vi "fgm_pipeline_partial_N22.vi"(6 "du_max":fxp<+/-,18,1>, 8 "x_vec":T3=[0.0, 0.0, 0.0, 0.0, 0.0, 0.0, 0.0, 0.0, 0.0, 0.0, 0.0, 0.0, 0.0, 0.0, 0.0, 0.0, 0.0, 0.0, 0.0, 0.0, 0.0, 0.0, 0.0, 0.0, 0.0], 11 "QP_params":T4={"maxIter"=0, "nuN"=24, "Ns_mpc"=0, "-beta"=-0.9987945556640625, "beta+1"=1.9987945556640625}) -> (0 "z":T1, 1 "delta u(k)":fxp<+/-,32,3>, 4 "y":T1)   [LabVIEW 2017]
uses:
  quadProgParams_pipe.ctl
  x_vec_type_pipe.ctl
  x_qp_scalar.ctl
  ziyi_pipe.ctl
  xtype_scalar.ctl
  <vilib>/rvi/Emulation/niFpgaEmulationIsFPGAContextNoSignature.vi
  <vilib>/rvi/DataTransferAndStorage/Container/Common/niFpgaContainerGetUniqueNameForEmu.vi
  <vilib>/rvi/Memory/Memory_Emulation/niFpgaMemoryEmulationCacheClearOnFirstRun.vi
  <vilib>/rvi/Memory/Memory_Emulation/nirvimemoryEmulationManagerCache_MakeExclusive.vi
  <vilib>/rvi/Memory/Memory_Emulation/niFpgaMemoryEmulationValidateCache.vi
  <vilib>/rvi/Memory/Memory_Emulation/nirvimemoryEmulationManagerCache_InsertValue.vi
  <vilib>/Utility/error.llb/Clear Errors.vi
  <vilib>/rvi/Memory/Memory_Emulation/nirvimemoryEmulationManagerCache_ReleaseExclusive.vi
  <vilib>/rvi/Memory/Memory_Emulation/nirvimemoryEmulationManagerCache_GetValue.vi
  <vilib>/rvi/Memory/Memory_Emulation/nirvimemoryEmulationManagerCache_SetValue.vi
  <vilib>/rvi/Emulation/niFpgaProcessEmulError.vi
  <vilib>/rvi/Emulation/niFpgaSctlEmulationGetInTimedLoop.vi
  <vilib>/rvi/DataTransferAndStorage/Container/XNode/niFpgaContainer.xnode
  <vilib>/rvi/DataTransferAndStorage/Register/Emulation/niFpgaRegisterEmulation.vi
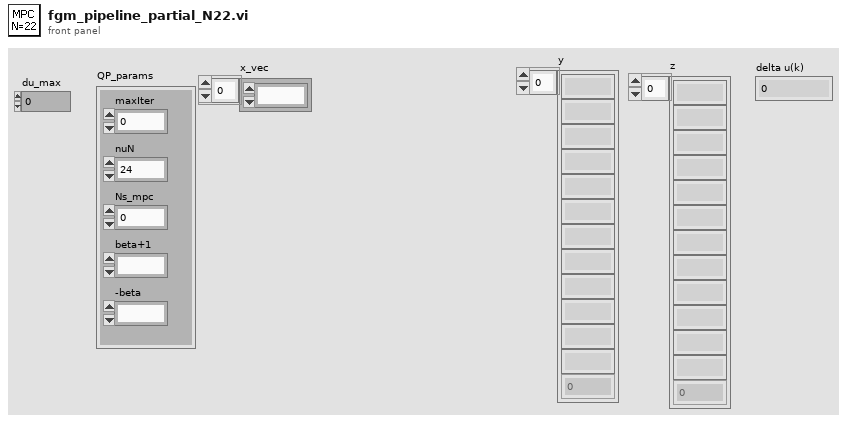
[diagram p1: front panel]
types:
  T1 = typedef "ziyi_pipe.ctl" = T2[]
  T2 = typedef "x_qp_scalar.ctl" = fxp<+/-,32,6>
  T3 = typedef "x_vec_type_pipe.ctl" = T2[]
  T4 = typedef "quadProgParams_pipe.ctl" = cluster{"maxIter":u16, "nuN":u16, "Ns_mpc":u16, "-beta":fxp<+/-,18,2>, "beta+1":fxp<+/-,18,2>}
  T5 = typedef "xtype_scalar.ctl" = fxp<+/-,32,6>
  T6 = typedef "ziyi_pipe_N22.ctl" = T2[]
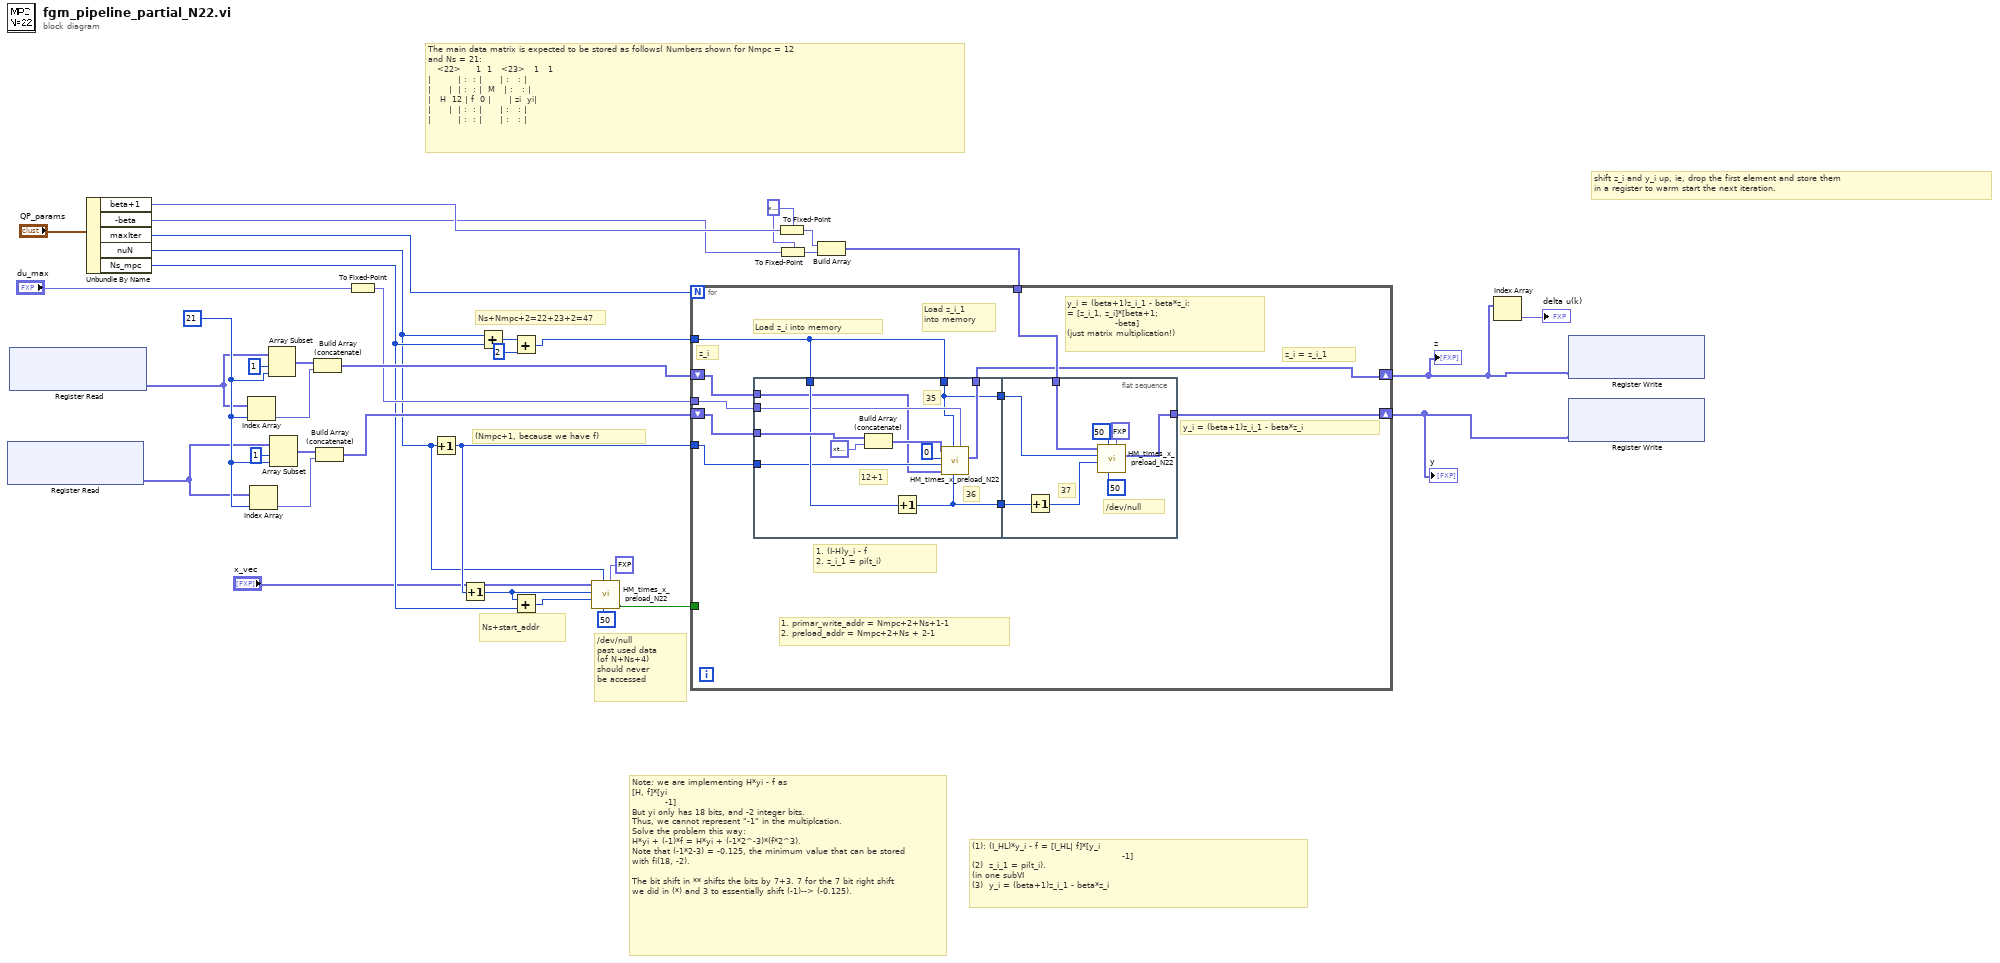
[diagram p0: block diagram]
diagram:
  w12 = 21 ("length")
  w19 = T5 0.0 ("xtype")
  # "The main data matrix is expected to be stored as follows( Numbers shown for Nmpc = 12\nand Ns = 21:\n   <22>     1  1   <23>   1   1\n|         | :  : |      | :   : |\n|      |  | :  : |  M   | :   : |\n|   H  12 | f  0 |      | zi  yi|\n|      |  | :  : |      | :   : |\n|         | :  : |      | :   : |"
  # "Ns+Nmpc+2=22+23+2=47"
  # "Ns+start_addr"
  # "(Nmpc+1, because we have f)"
  # "/dev/null\npast used data\n(of N+Ns+4)\nshould never\nbe accessed"
  # "Note: we are implementing H*yi - f as\n[H, f]*[yi\n           -1]\nBut yi only has 18 bits, and -2 integer bits. \nThus, we cannot represent \"-1\" in the multiplcation.\nSolve the problem this way:\nH*yi + (-1)*f = H*yi + (-1*2^-3)*(f*2^3).\nNote that (-1*2-3) = -0.125, the minimum value that can be stored\nwith fi(18, -2).\n\nThe bit shift in ** shifts the bits by 7+3. 7 for the 7 bit right shift\nwe did in (*) and 3 to essentially shift (-1)--> (-0.125)."
  # "(1): (I_HL)*y_i - f = [I_HL| f]*[y_i\n                                                  -1]\n(2)  z_i_1 = pi(t_i).\n(in one subVI\n(3)  y_i = (beta+1)z_i_1 - beta*z_i"
  # "shift z_i and y_i up, ie, drop the first element and store them\nin a register to warm start the next iteration."
  n1 = xnode ("Register Read")() -> ("Data"=w9:fxp<+/-,32,6>[])  [unwired: 1 in, 1 out]
  n2 = xnode ("Register Read")() -> ("Data"=w8:fxp<+/-,32,6>[])  [unwired: 1 in, 1 out]
  n3 = Unbundle By Name("QP_params") -> ("beta+1"=w34:fxp<+/-,18,2>, "-beta"=w33:fxp<+/-,18,2>, "maxIter"=w35:u16, "nuN"=w7:u16, "Ns_mpc"=w16:u16)
  n4 = Index Array(array=w8, index=w12) -> (element=w22:fxp<+/-,32,6>)
  n5 = Index Array(array=w9, index=w12) -> (element=w23:fxp<+/-,32,6>)
  n6 = Array Subset(array=w8, index=1, length=w12) -> (w26:fxp<+/-,32,6>[])
  n7 = Array Subset(array=w9, index=1, length=w12) -> (w24:fxp<+/-,32,6>[])
  n8 = Build Array (concatenate)(w26, w22) -> (w21:fxp<+/-,32,6>[])
  n9 = Build Array (concatenate)(w24, w23) -> (w20:fxp<+/-,32,6>[])
  n10 = To Fixed-Point(number="du_max") -> (fixed-point=w18:fxp<+/-,18,5>)  [unwired: 1 in]
  n11 = Increment(x=w7) -> (x+1=w29:u16)
  n12 = Increment(x=w29) -> (x+1=w2:u16)
  n13 = Add(x=w7, y=w16) -> (x+y=w15:u16)
  n14 = Add(x=w15, y=u16 2) -> (x+y=w13:u16)
  n15 = Add(x=w2, y=w16) -> (x+y=w1:u16)
  n16 = call "HM_times_x_preload_N22.vi"("SLMAX"=fxp<+/-,18,5> 15.9998779296875, "preload_addr"=u8 50, "primary_write_addr"=w7, "Ns+StartIndex"=w1, "StartIndex"=w2, "x_vec"="x_vec") -> ("done"=w5:bool)  [unwired: 4 in, 1 out]
  n17 = To Fixed-Point(fixed-point type=w19, number=w34) -> (fixed-point=w32:T5)
  n18 = To Fixed-Point(fixed-point type=w19, number=w33) -> (fixed-point=w31:T5)
  n19 = Build Array(w32, w31) -> (w30:T5[])
  n20 = for {
    N: w35 -> [_]
    shift-right: [w45] -> w10
    shift-left: w20 -> [w44]
    shift-right: [w41] -> w11
    shift-left: w21 -> [w40]
    tunnel: w30 -> [w46]
    tunnel: w18 -> [w42]
    tunnel: w5 -> [_]
    tunnel: w29 -> [w43]
    tunnel: w13 -> [w38]
    # "1. primar_write_addr = Nmpc+2+Ns+1-1\n2. preload_addr = Nmpc+2+Ns + 2-1"
    # "y_i = (beta+1)z_i_1 - beta*z_i:\n= [z_i_1, z_i]*[beta+1;\n                -beta]\n(just matrix multiplication!)"
    # "Load z_i into memory"
    # "Load z_i_1\ninto memory"
    # "1. (I-H)y_i - f\n2. z_i_1 = pi(t_i)"
    # "z_i = z_i_1"
    # "y_i = (beta+1)z_i_1 - beta*z_i"
    # "z_i"
    n21 = flat-sequence {
      tunnel: w40 -> [w47]
      tunnel: w44 -> [w57]
      tunnel: w43 -> [w48]
      tunnel: w42 -> [w52]
      tunnel: [w53] -> w41
      tunnel: w38 -> [w51]
      tunnel: [w51] -> w39
      tunnel: w38 -> [w55]
      tunnel: [w50] -> w37
      tunnel: w46 -> [w60]
      tunnel: [w64] -> w45
      tunnel: w39 -> [w61]
      tunnel: w37 -> [w65]
      frame #0 {
        # "35"
        # "36"
        # "12+1"
        n22 = Build Array (concatenate)(w57, T5 -1.0 ("xtype")) -> (w54:T5[])
        n23 = Increment(x=w55) -> (x+1=w50:u16)
        n24 = call "HM_times_x_preload_N22.vi"("SLMAX"=w52, "preload_addr"=w50, "primary_write_addr"=w51, "preload_vec"=w47, "Ns+StartIndex"=w48, "StartIndex"=u8 0 ("rowOffset"), "x_vec"=w54) -> ("A*x"=w53:T6)  [unwired: 3 in, 1 out]
      }
      frame #1 {
        # "37"
        # "/dev/null"
        n25 = Increment(x=w65) -> (x+1=w62:u16)
        n26 = call "HM_times_x_preload_N22.vi"("SLMAX"=fxp<+/-,18,5> 15.9998779296875, "preload_addr"=u8 50, "primary_write_addr"=u8 50, "Ns+StartIndex"=w62, "StartIndex"=w61, "x_vec"=w60) -> ("A*x"=w64:T6)  [unwired: 4 in, 1 out]
      }
    }
  }
  "y" <- w10
  "z" <- w11
  n27 = Index Array(array=w11) -> (element=→"delta u(k)":T2)  [unwired: 1 in]
  n28 = xnode ("Register Write")("Data"=w11) -> ()  [unwired: 1 in, 1 out]
  n29 = xnode ("Register Write")("Data"=w10) -> ()  [unwired: 1 in, 1 out]
